vi "write keyword - string.vi"(8 "error in (no error)":errorcluster, 9 "value":string, 10 "keyword":string, 11 "Simulated_Header in":refnum<class "Simulated_Header.lvclass">) -> (0 "error out":errorcluster, 3 "Simulated_Header out":refnum<class "Simulated_Header.lvclass">)   [LabVIEW 2018, in "Simulated_Header.lvclass"]
uses:
  Simulated_Header.lvclass
  Simulated_Header.lvclass/Simulated_Header.ctl
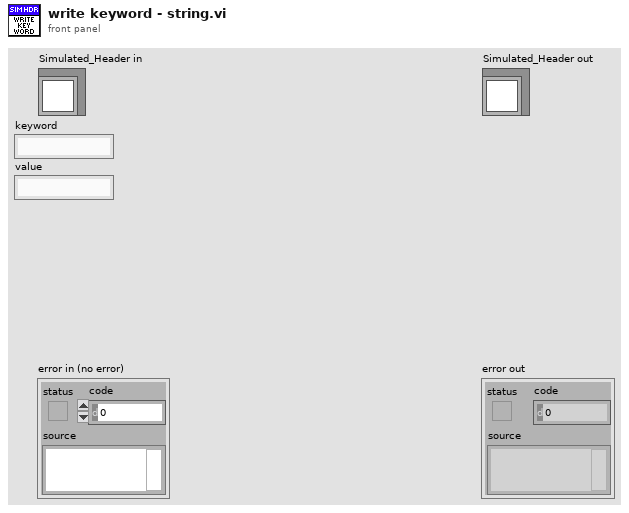
[diagram p1: front panel]
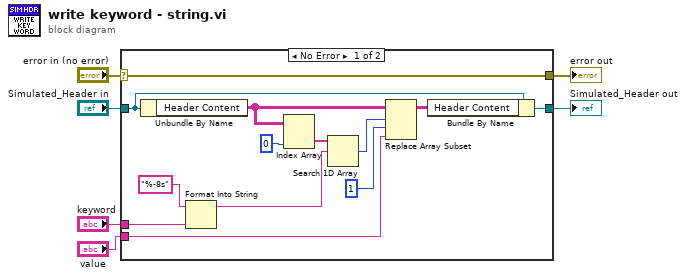
[diagram p0: block diagram]
diagram:
  n1 = case shown="No Error" "error in (no error)" {
    selector: "error in (no error)" -> [w19 w21]
    tunnel: [w19 w21] -> w5
    tunnel: [w11 w20] -> w3
    tunnel: "Simulated_Header in" -> [w12 w20]
    tunnel: "keyword" -> [w9 _]
    tunnel: "value" -> [w13 _]
    frame No Error {
      n2 = Unbundle By Name(w12) -> ("Header Content"=w16:string[][])
      n3 = Format Into String(format string="%-8s", w9) -> (resulting string=w8:string)  [unwired: 2 in, 1 out]
      n4 = Index Array(array=w16, index (col)=0 ("disabled index (col)")) -> (element=w17:string[])  [unwired: 1 in]
      n5 = Search 1D Array(1D array=w17, element=w8) -> (index of element=w14:i32)  [unwired: 1 in]
      n6 = Replace Array Subset(array=w16, new element=w13, index (row)=w14, index (col)=1 ("disabled index (col)")) -> (w10:string[][])
      n7 = Bundle By Name(cluster=w12, "Header Content"=w10) -> (w11:refnum<class "Simulated_Header.lvclass">)
    }
    frame Error {
    }
  }
  "error out" <- w5
  "Simulated_Header out" <- w3
